vi "Engineering mode.vi"() -> ()   [LabVIEW 2017]
uses:
  Ctrls/TesterInfo.ctl
  Ctrls/control_hard.ctl
  Ctrls/AllControls.ctl
  Ctrls/Position Config.ctl
  Ctrls/HD Config.ctl
  <vilib>/Utility/miscctls.llb/LVRowAndColumnTypeDef.ctl
  ComVIS/Files/Ini/WriteIniFiles_ByVarient.vi
  <vilib>/Utility/file.llb/Write Delimited Spreadsheet (string).vi
  HardWare/ADLINK/IO/Adlink IO/Adlink IO.lvlib
  <instrlib>/GPP/GPP.lvlib
panel:
  out "URAT.COM":refnum<visa-resource-name>
  in  "Production Mode":bool
  out "Boolean":bool=TRUE
  in  "Data":string
  out "Size":i32
  in  "AllControls":T1
  out "Save_status":string
  in  "Selecttion":T2(tab)
  in  "HD Config":T3
  in  "HD Config Save":bool
  in  "SW Config Save":bool
  in  "TesterInfo":T4
  in  "Table":T5(tab)
  in  "Table_Data":string[][](table)
  in  "Title_Data":string[][](table)
  in  "Config":string[][](table)
  in  "SKU_Table":string[][](table)
  in  "Debug":T6
  in  "IO":i32(listbox)
  in  "Reset":bool
  in  "Position Config":T7
  in  "Position Config Save":bool
  in  "NFC":bool
  out "NFC Data":string
  in  "Voltage":dbl min=0.0 max=25.0
  in  "Current":dbl min=0.0 max=48.0
  in  "Read Current&Voltage":bool
  out "ERROR":string
  in  "Write Current&Voltage":bool
  out "Read Current  (A)":dbl
  out "Read Voltage  (V)":dbl
  in  "Set Current  (A)":dbl=1.0
  in  "Set Voltage  (V)":dbl=3.7
  # "Unit: mm"
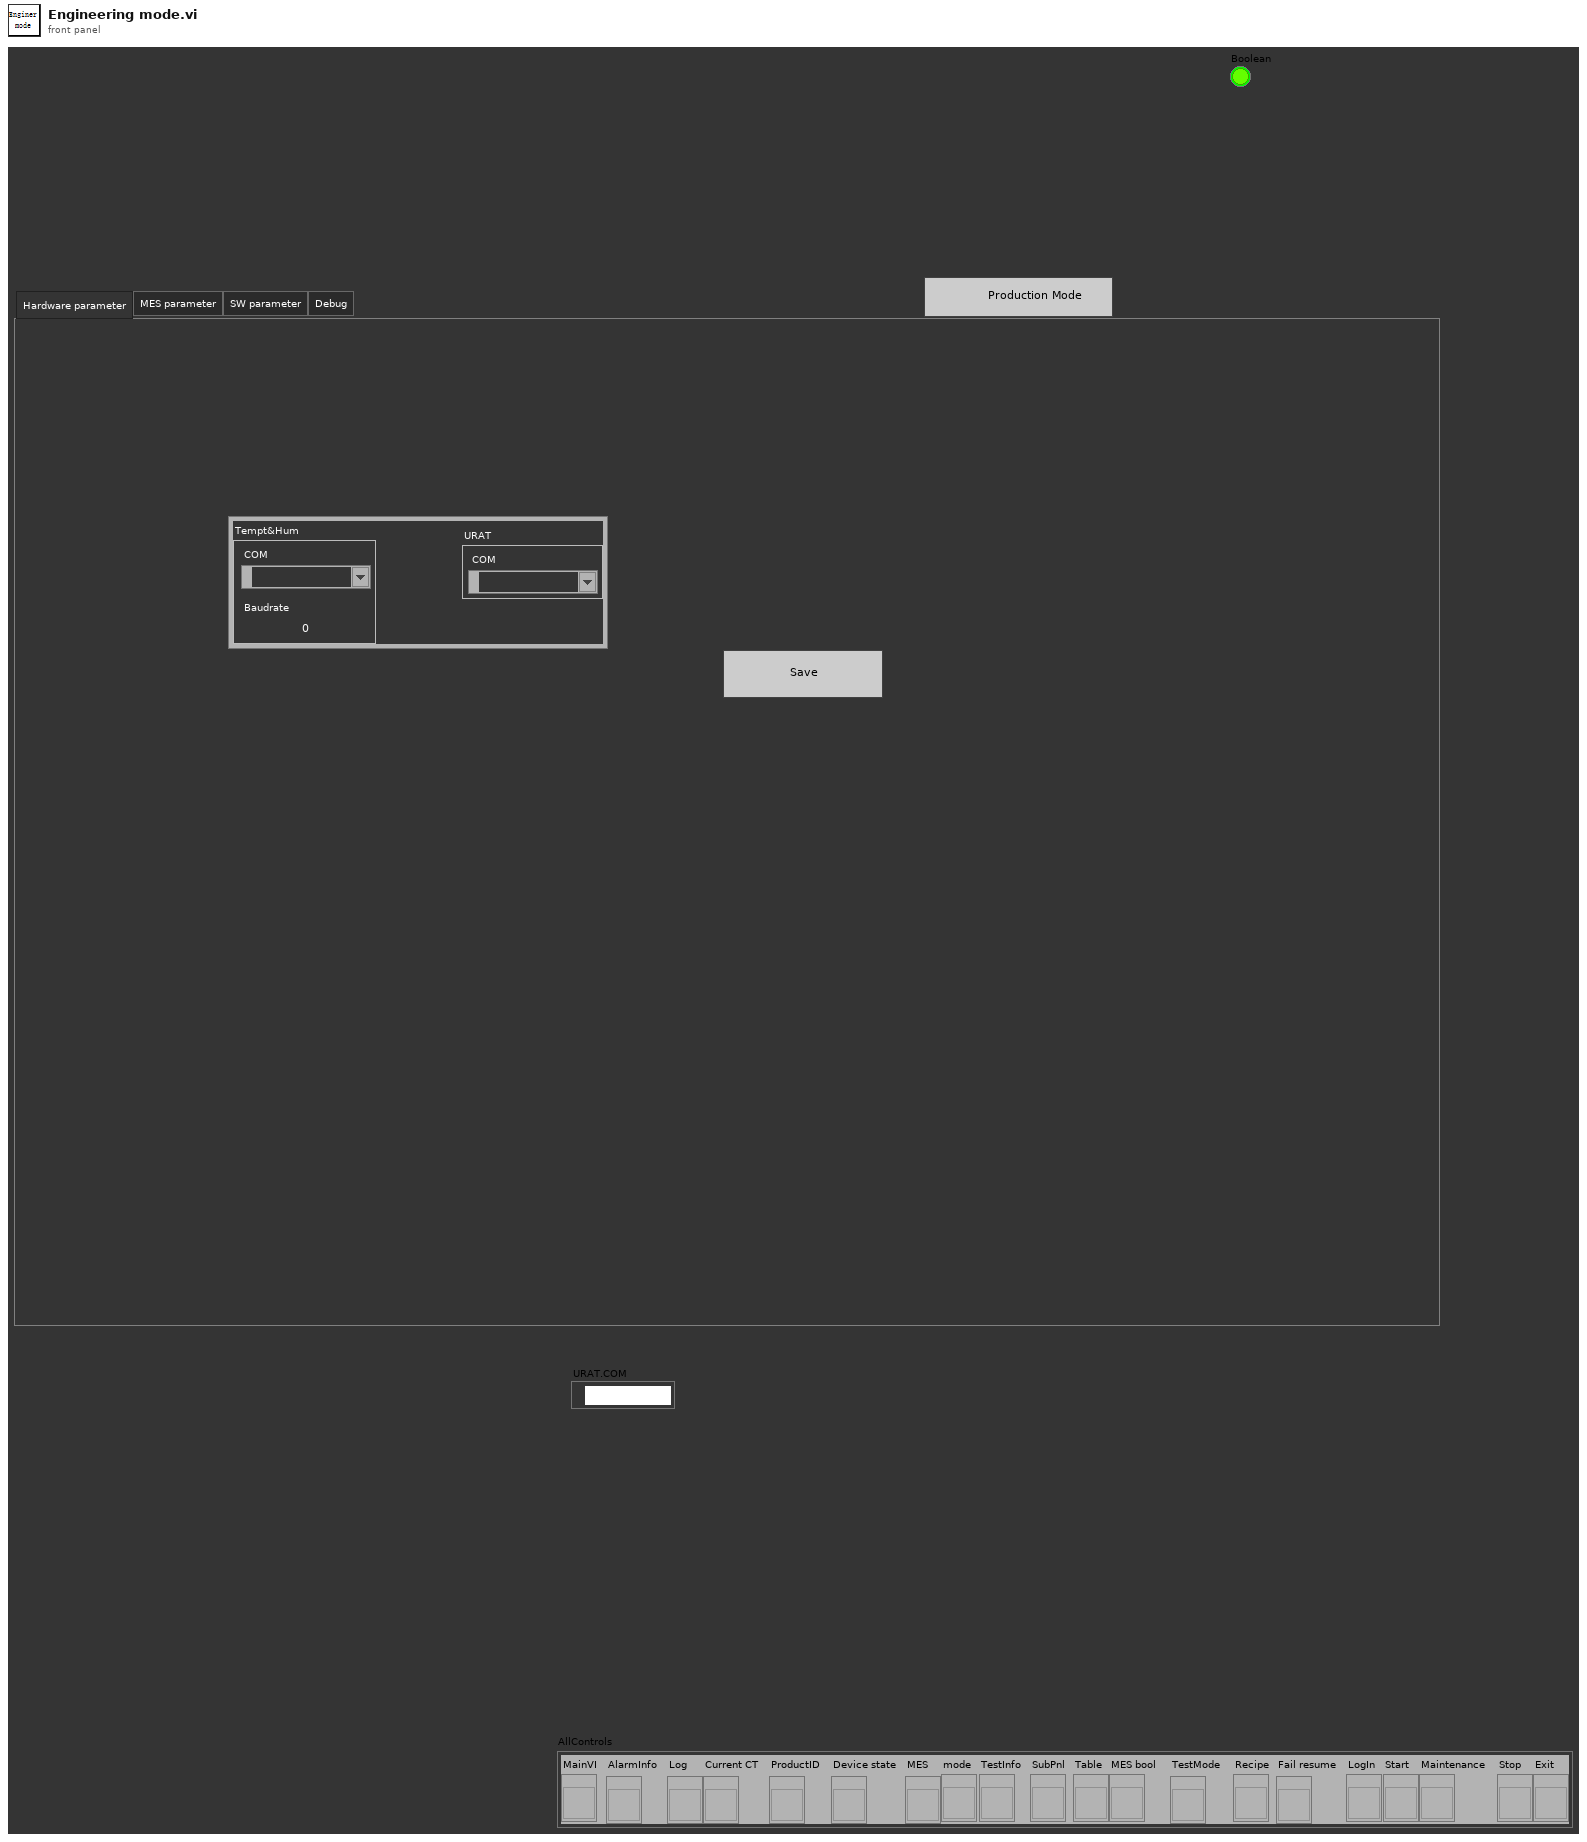
[diagram p1: front panel]
types:
  T1 = typedef "AllControls.ctl" = cluster{"MainVI":refnum<vi>, "AlarmInfo":refnum<vi>, "Log":refnum<vi>, "Current CT":refnum<vi>, "ProductID":refnum<vi>, "Device state":refnum<vi>, "MES":refnum<vi>, "mode":refnum<vi>, "TestInfo":refnum<vi>, "SubPnl":refnum<vi>, "Table":refnum<vi>, "MES bool":refnum<vi>, "TestMode":refnum<vi>, "Recipe":refnum<vi>, "Fail resume":refnum<vi>, "LogIn":refnum<vi>, "Start":refnum<vi>, "Maintenance":refnum<vi>, "Stop":refnum<vi>, "Exit":refnum<vi>}
  T2 = enum32{"Hardware parameter", "MES parameter", "SW parameter", "Debug"}
  T3 = typedef "HD Config.ctl" = cluster{" PC":cluster{"PC Address":u8[], "PC Port":i32}, "FCO":cluster{"COM":refnum<visa-resource-name>, "Baudrate":u32}, "DC Power ":cluster{"COM":refnum<visa-resource-name>, "Baudrate":u32}, "PW3336":cluster{"COM":refnum<visa-resource-name>, "Baudrate":u32}, "Lefoo":cluster{"COM":refnum<visa-resource-name>, "Baudrate":u32}, "Tempt&Hum":cluster{"COM":refnum<visa-resource-name>, "Baudrate":u32}, "DIPC":cluster{"COM":refnum<visa-resource-name>}, "Daemon":cluster{"IP Address":string, "Port":u16, "Retry":u16}, "URAT":cluster{"COM":refnum<visa-resource-name>, "Baudrate":u32}, "Fail_resume_mode":bool, "GRR":bool}
  T4 = typedef "TesterInfo.ctl" = cluster{"Station Name":string, "Station Code":string, "ES NO.":string, "Tester ID":string, "PassMark Revision":string, "Rig ID":string, "Deamon_vision":string, "Project Name":string, "FFTesterPath":path, "Enable_User":bool, "Mode":enum16{"682"}, "MES":bool}
  T5 = enum32{"Process_parameter_Setting", "Passmark_Setting", "Setting_Config", "SKU_Table"}
  T6 = typedef "control_hard.ctl" = enum32{"IO Control", "Motor_Plate control", "Led Read", "NFC ", "PW3336_Power Meter", "Lefoo_Atm Pressure", "Power Supply", "Set EOL_URAT"}
  T7 = typedef "Position Config.ctl" = cluster{"OrificeSize_12.7":i32, "OrificeSize_13":i32, "OrificeSize_30":i32, "OrificeSize_16":i32}
  T8 = cluster{"COM":refnum<visa-resource-name>, "Baudrate":u32}
  T9 = cluster{"DI dev":i32[], "DI line":i32[], "Port":i32[], "DO dev":i32[], "DO line":i32[], "IO Data":string[][], "IO f":i16[]}
  T10 = typedef "amc_Message Queue.ctl" = refnum<queue>
  T11 = typedef "LVRowAndColumnTypeDef.ctl" = cluster{"Row":i32, "Column":i32}
  T12 = typedef "LVPoint32TypeDef.ctl" = cluster{"Horizontal":i32, "Vertical":i32}
  T13 = enum8{"Enabled", "Disabled", "Disabled and Grayed Out"}
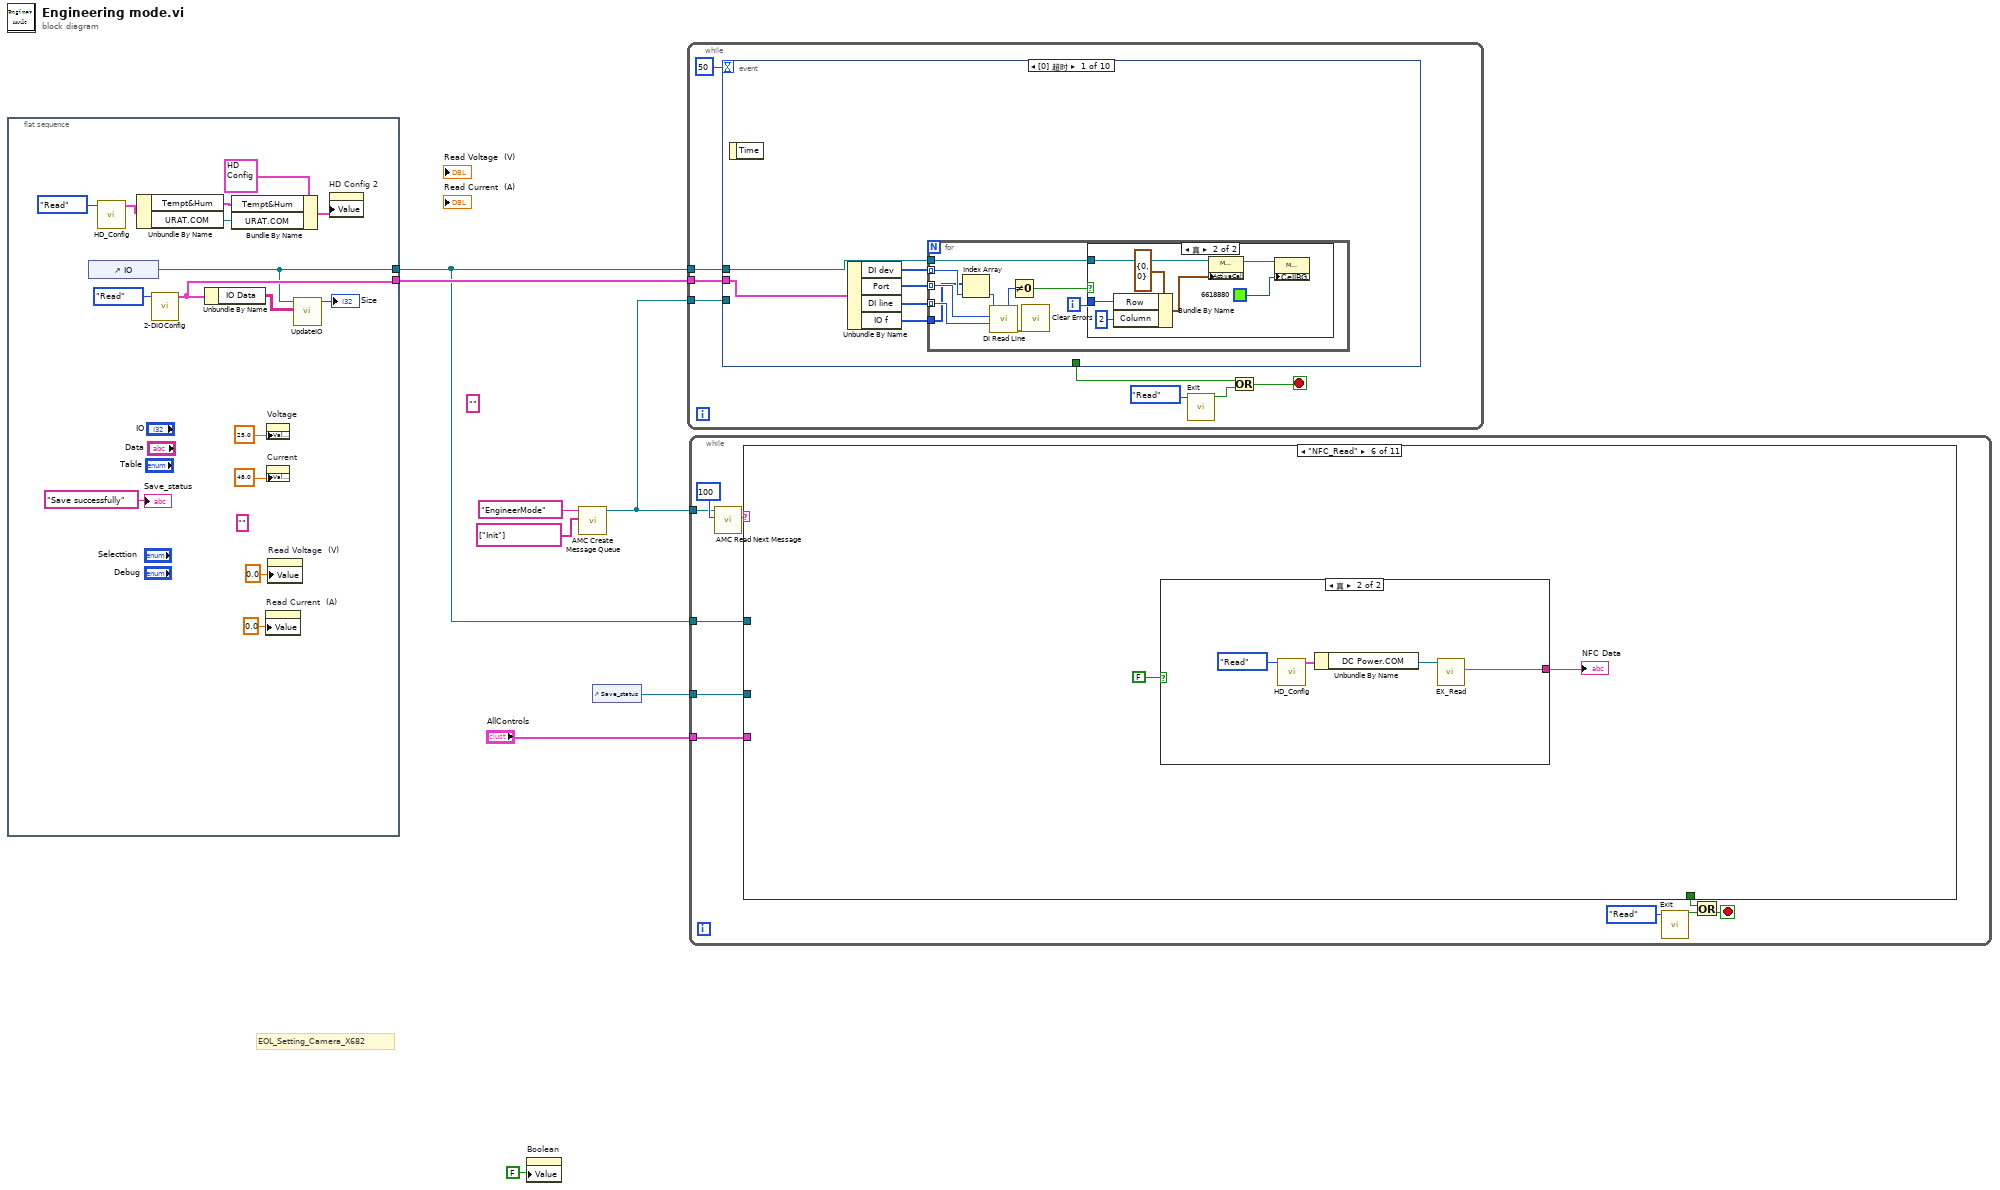
[diagram p0: block diagram]
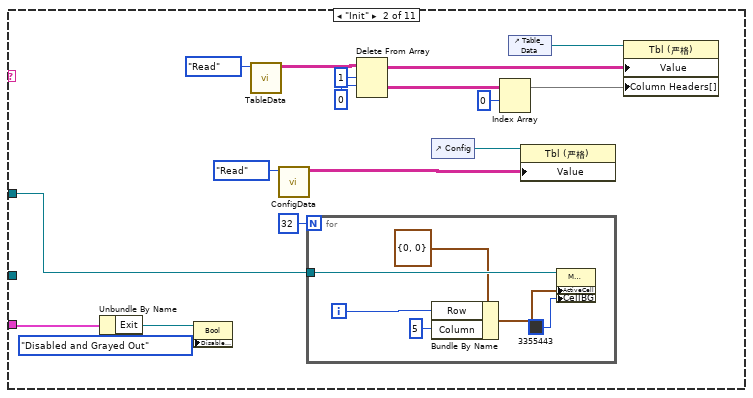
[diagram p3: hidden frame]
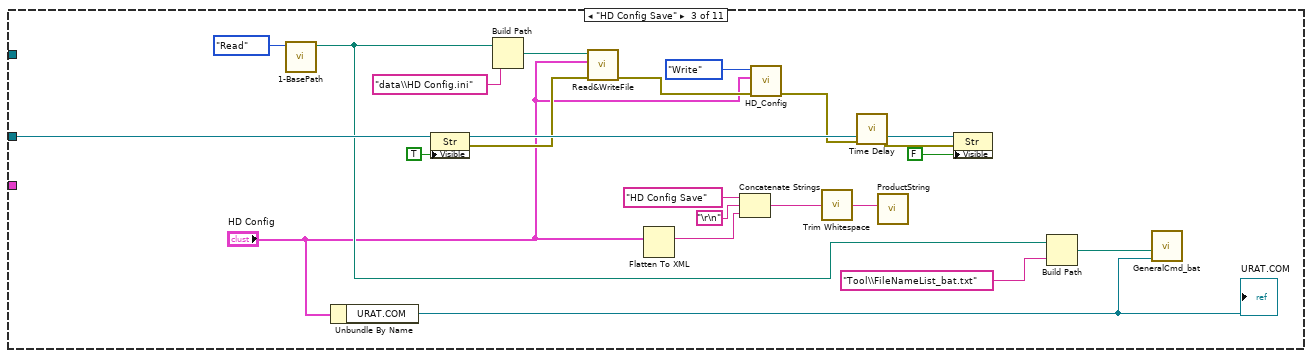
[diagram p4: hidden frame]
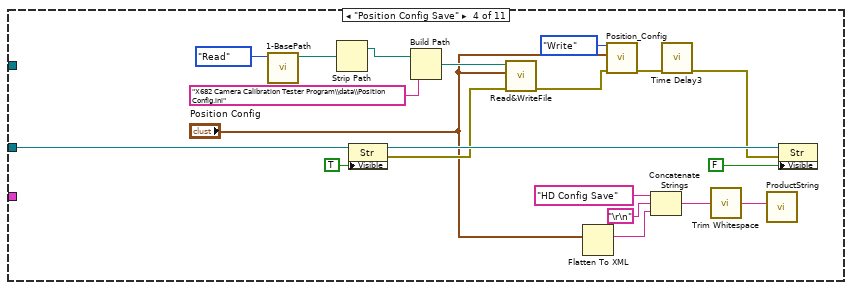
[diagram p5: hidden frame]
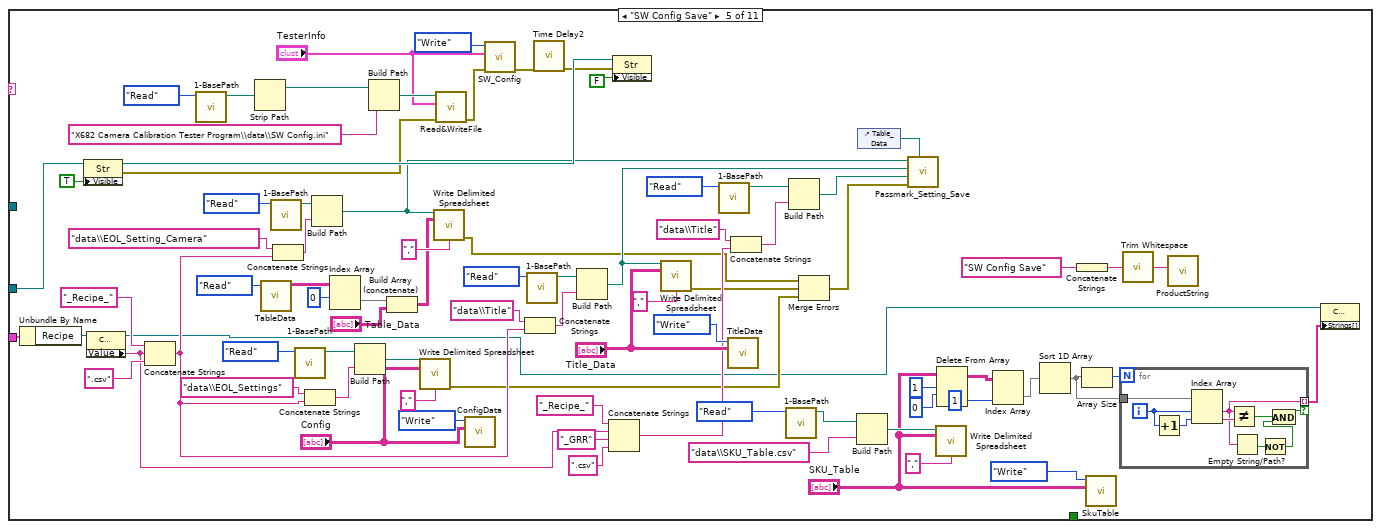
[diagram p6: hidden frame]
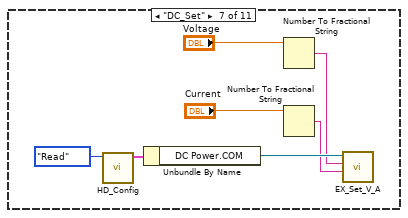
[diagram p8: hidden frame]
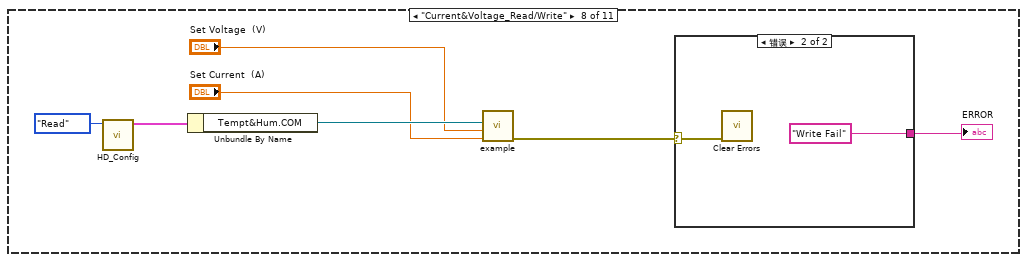
[diagram p9: hidden frame]
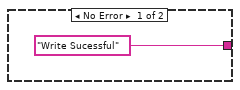
[diagram p10: hidden frame]
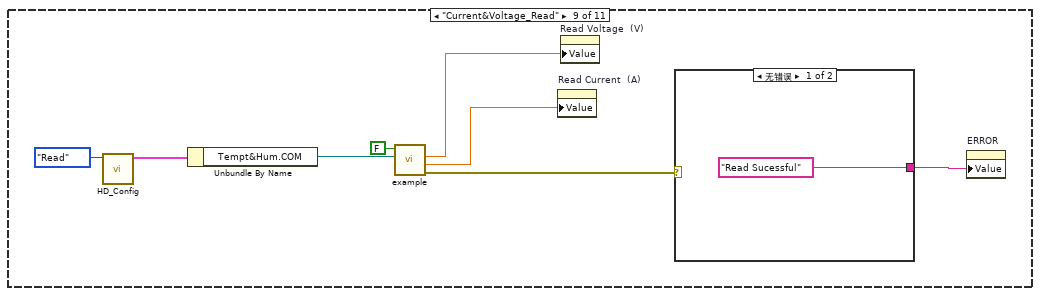
[diagram p11: hidden frame]
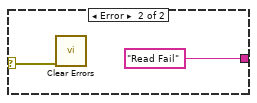
[diagram p12: hidden frame]
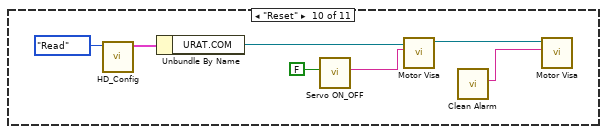
[diagram p13: hidden frame]
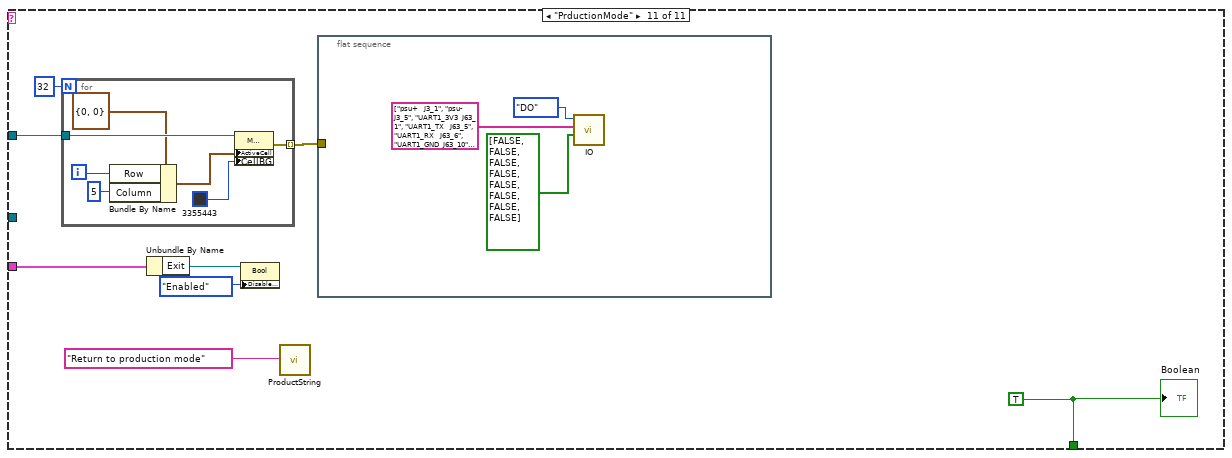
[diagram p14: hidden frame]
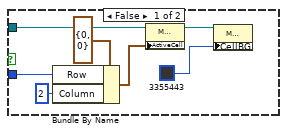
[diagram p15: hidden frame]
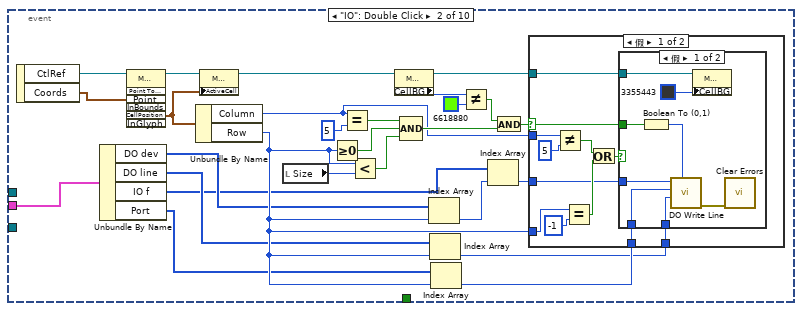
[diagram p16: hidden frame]
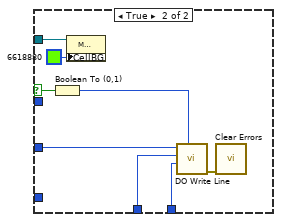
[diagram p18: hidden frame]
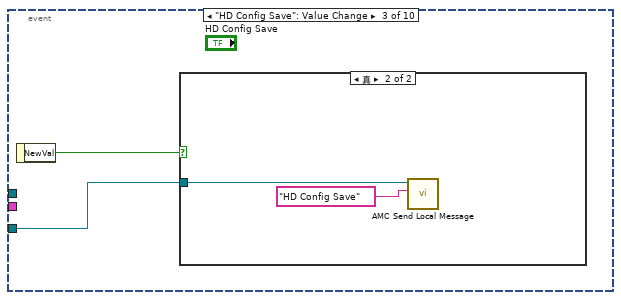
[diagram p19: hidden frame]
diagram:
  (unwired) "" ("concatenated string")
  # "EOL_Setting_Camera_X682"
  n1 = flat-sequence {
    tunnel: [w23] -> w3
    tunnel: [w21] -> w2
    frame #0 {
      (unwired) "" ("Data Return")
      n2 = control-ref of="IO"() -> (w21:refnum<vi>)
      n3 = call "HD_Config.vi"("Step"=enum16{"Initial", "Write", "Read"}."Read") -> ("HD Config out"=w17:T3)  [unwired: 9 in, 1 out]
      n4 = Unbundle By Name(w17) -> ("Tempt&Hum"=w14:T8, "URAT.COM"=w10:refnum<visa-resource-name>)
      n5 = call "2-DIOConfig.vi"("Step"=enum16{"Initial", "Write", "Read"}."Read") -> ("DIO pra out"=w23:T9)  [unwired: 9 in, 1 out]
      n6 = Unbundle By Name(w23) -> ("IO Data"=w22:string[][])
      n7 = Bundle By Name(cluster=T3 {" PC"={"PC Address"=[], "PC Port"=0}, "FCO"={"COM"="", "Baudrate"=0}, "DC Power "={"COM"="", "Baudrate"=0}, "PW3336"={"COM"="", "Baudrate"=0}, "Lefoo"={"COM"="", "Baudrate"=0}, "Tempt&Hum"={"COM"="", "Baudrate"=0}, "DIPC"={"COM"=""}, "Daemon"={"IP Address"="", "Port"=0, "Retry"=0}, "URAT"={"COM"="", "Baudrate"=0}, "Fail_resume_mode"=FALSE, "GRR"=FALSE} ("HD Config 2"), "Tempt&Hum"=w14, "URAT.COM"=w10) -> (w13:T3)
      n8 = property on="Read Current  (A)" class="DigNum (严格)"("Value"=0.0 ("Read Current")) -> ()  [unwired: 2 in, 2 out]
      n9 = property on="Voltage" class="DigNum (strict)"("Value"=25.0 ("Voltage")) -> ()  [unwired: 2 in, 2 out]
      n10 = property on="Current" class="DigNum (strict)"("Value"=48.0 ("Current")) -> ()  [unwired: 2 in, 2 out]
      n11 = property on="Read Voltage  (V)" class="DigNum (严格)"("Value"=0.0 ("Read Voltage")) -> ()  [unwired: 2 in, 2 out]
      n12 = call "UpdateIO.vi"("IO Data"=w22, "MulticolumnListbox输入"=w21) -> ("大小"=→"Size":i32)  [unwired: 9 in]
      n13 = property on="HD Config 2" class="Clust (严格)"("Value"=w13) -> ()  [unwired: 2 in, 2 out]
      "Save_status" <- "Save successfully" ("Save_status")
    }
  }
  n14 = property on="Boolean" class="Bool (严格)"("Value"=FALSE ("Boolean")) -> ()  [unwired: 2 in, 2 out]
  n15 = call "AMC Create Message Queue.vi"("Initial Message Names"=string[] ["Init"], "Message Queue Name"="EngineerMode" ("Message queue name (unnamed)")) -> ("Message Queue out"=w7:T10)  [unwired: 3 in, 6 out]
  n16 = control-ref of="Save_status"() -> (w6:refnum<vi>)
  n17 = while {
    tunnel: w7 -> [w29]
    tunnel: w2 -> [w27]
    tunnel: w3 -> [w26]
    stop <- w25 stop-if-true
    n18 = event shown="[0] 超时" {
      selector: _ -> [_ _ _ _ _ _ _ _ _ _]
      dyn-events: _ -> [_ _ _ _ _ _ _ _ _ _]
      timeout: 50 -> [_ _ _ _ _ _ _ _ _ _]
      tunnel: w29 -> [_ _ w119 w122 w127 w132 w139 w143 w146 w151]
      tunnel: [_ _ _ _ _ _ _ _ _ w150] -> w28
      tunnel: w27 -> [w33 _ _ _ _ _ _ _ _ _]
      tunnel: w26 -> [w34 w65 _ _ _ _ _ _ _ _]
      event Timeout {
        n19 = event-data() -> ()  [unwired: 1 in, 1 out]
        n20 = Unbundle By Name(w34) -> ("DI dev"=w35:i32[], "Port"=w36:i32[], "DI line"=w37:i32[], "IO f"=w38:i16[])
        n21 = for {
          tunnel: w33 -> [w44]
          tunnel: w35 -> [w41] mode=indexing
          tunnel: w37 -> [w45] mode=indexing
          tunnel: w36 -> [w42] mode=indexing
          tunnel: w38 -> [w39]
          i -> [w43]
          n22 = Index Array(array=w39, index=w41) -> (element=w40:i16)
          n23 = call "DI Read Line.vi"("Line"=w45, "Port"=w42, "CardNumber"=w40) -> ("error out"=w48:errorcluster, "State out"=w47:u16)  [unwired: 6 in, 1 out]
          n24 = Not Equal To 0?(x=w47) -> (x != 0?=w46:bool)
          n25 = call <vilib>:"Clear Errors.vi"("error in (no error)"=w48) -> ()  [unwired: 5 in, 2 out]
          n26 = case shown="真" w46 {
            tunnel: w43 -> [w50 w59]
            tunnel: w44 -> [w49 w56]
            frame False {
              n27 = Bundle By Name(cluster=T11 {"Row"=0, "Column"=0} ("活动单元格:活动单元格"), "Row"=w50, "Column"=2) -> (w53:T11)
              n28 = property class="MCListbox (严格)"(reference=w49, "ActiveCell"=w53) -> (reference out=w55:refnum<vi>)  [unwired: 1 in, 1 out]
              n29 = property class="MCListbox (严格)"(reference=w55, "CellBG"=u32 3355443) -> ()  [unwired: 1 in, 2 out]
            }
            frame True {
              n30 = Bundle By Name(cluster=T11 {"Row"=0, "Column"=0} ("活动单元格:活动单元格"), "Row"=w59, "Column"=2) -> (w60:T11)
              n31 = property class="MCListbox (严格)"(reference=w56, "ActiveCell"=w60) -> (reference out=w62:refnum<vi>)  [unwired: 1 in, 1 out]
              n32 = property class="MCListbox (严格)"(reference=w62, "CellBG"=u32 6618880) -> ()  [unwired: 1 in, 2 out]
            }
          }
        }
      }
      event "IO": Double Click {
        n33 = event-data() -> ("CtlRef"=w64:refnum<vi>, "Coords"=w63:T12)  [unwired: 1 in]
        n34 = Unbundle By Name(w65) -> ("DO dev"=w70:i32[], "DO line"=w69:i32[], "IO f"=w68:i16[], "Port"=w87:i32[])
        n35 = invoke class="MCListbox (严格)" method="Point To Row Column"(reference=w64, "Point"=w63) -> (reference out=w83:refnum<vi>, "CellPosition"=w74:T11)  [unwired: 5 in, 5 out]
        n36 = Unbundle By Name(w74) -> ("Column"=w71:i32, "Row"=w88:i32)
        n37 = property class="MCListbox (严格)"(reference=w83, "ActiveCell"=w74) -> (reference out=w82:refnum<vi>)  [unwired: 1 in, 1 out]
        n38 = local read "Size"() -> (w73:i32)
        n39 = Greater Or Equal To 0?(x=w88) -> (x >= 0?=w79:bool)
        n40 = Equal?(x=w71, y=5) -> (x = y?=w80:bool)
        n41 = Less?(x=w88, y=w73) -> (x < y?=w72:bool)
        n42 = property class="MCListbox (严格)"(reference=w82) -> (reference out=w75:refnum<vi>, "CellBG"=w77:u32)  [unwired: 1 in, 1 out]
        n43 = Compound Arithmetic op=AND(w80, w79, w72) -> (w81:bool)
        n44 = Index Array(array=w70, index=w88) -> (element=w84:i32)
        n45 = Index Array(array=w69, index=w88) -> (element=w86:i32)
        n46 = Index Array(array=w87, index=w88) -> (element=w89:i32)
        n47 = Not Equal?(x=w77, y=u32 6618880) -> (x != y?=w78:bool)
        n48 = Index Array(array=w68, index=w84) -> (element=w85:i16)
        n49 = And(x=w78, y=w81) -> (x .and. y?=w76:bool)
        n50 = case shown="假" w76 {
          selector: w76 -> [w98 w113]
          tunnel: w75 -> [w101 w117]
          tunnel: w71 -> [w97 _]
          tunnel: w85 -> [w92 w115]
          tunnel: w86 -> [w91 w114]
          tunnel: w88 -> [w93 _]
          tunnel: w89 -> [w90 w110]
          frame False {
            n51 = Not Equal?(x=w97, y=5) -> (x != y?=w94:bool)
            n52 = Equal?(x=w93, y=-1) -> (x = y?=w99:bool)
            n53 = Or(x=w94, y=w99) -> (x .or. y?=w95:bool)
            n54 = case shown="假" w95 {
              tunnel: w101 -> [w108 _]
              tunnel: w98 -> [w103 _]
              tunnel: w92 -> [w104 _]
              tunnel: w91 -> [w105 _]
              tunnel: w90 -> [w102 _]
              frame False {
                n55 = Boolean To (0,1)(Boolean=w103) -> (0, 1=w107:i16)
                n56 = call "DO Write Line.vi"("Value"=w107, "Line"=w105, "Port"=w102, "CardNumber"=w104) -> ("error out"=w106:errorcluster)  [unwired: 6 in, 1 out]
                n57 = property class="MCListbox (严格)"(reference=w108, "CellBG"=u32 3355443) -> ()  [unwired: 1 in, 2 out]
                n58 = call <vilib>:"Clear Errors.vi"("error in (no error)"=w106) -> ()  [unwired: 5 in, 2 out]
              }
              frame True {
              }
            }
          }
          frame True {
            n59 = Boolean To (0,1)(Boolean=w113) -> (0, 1=w112:i16)
            n60 = property class="MCListbox (严格)"(reference=w117, "CellBG"=u32 6618880) -> ()  [unwired: 1 in, 2 out]
            n61 = call "DO Write Line.vi"("Value"=w112, "Line"=w114, "Port"=w110, "CardNumber"=w115) -> ("error out"=w111:errorcluster)  [unwired: 6 in, 1 out]
            n62 = call <vilib>:"Clear Errors.vi"("error in (no error)"=w111) -> ()  [unwired: 5 in, 2 out]
          }
        }
      }
      event "HD Config Save": Value Change {
        n63 = event-data() -> ("NewVal"=w118:bool)  [unwired: 1 in]
        n64 = case shown="真" w118 {
          tunnel: w119 -> [_ w121]
          frame False {
          }
          frame True {
            n65 = call "AMC Send Local Message.vi"("Message Name"="HD Config Save", "Message Queue in"=w121) -> ()  [unwired: 8 in, 2 out]
          }
        }
      }
      event "SW Config Save": Value Change {
        n66 = event-data() -> ("NewVal"=w123:bool)  [unwired: 1 in]
        n67 = case shown="真" w123 {
          tunnel: w122 -> [_ w125]
          frame False {
          }
          frame True {
            n68 = call "AMC Send Local Message.vi"("Message Name"="SW Config Save", "Message Queue in"=w125) -> ()  [unwired: 8 in, 2 out]
          }
        }
      }
      event "Position Config Save": Value Change {
        n69 = event-data() -> ("NewVal"=w126:bool)  [unwired: 1 in]
        n70 = case shown="真" w126 {
          tunnel: w127 -> [_ w129]
          frame False {
          }
          frame True {
            n71 = call "AMC Send Local Message.vi"("Message Name"="Position Config Save", "Message Queue in"=w129) -> ()  [unwired: 8 in, 2 out]
          }
        }
      }
      event "Write Current&Voltage": Value Change {
        n72 = event-data() -> ("NewVal"=w131:bool)  [unwired: 1 in]
        n73 = case shown="真" w131 {
          tunnel: w132 -> [_ w133]
          frame False {
          }
          frame True {
            n74 = call "AMC Send Local Message.vi"("Message Name"="Current&Voltage_Read/Write", "Message Queue in"=w133) -> ()  [unwired: 8 in, 2 out]
          }
        }
        n75 = property on="ERROR" class="Str"("Value"="" ("ERROR")) -> ()  [unwired: 2 in, 2 out]
      }
      event "Read Current&Voltage": Value Change {
        n76 = event-data() -> ("NewVal"=w138:bool)  [unwired: 1 in]
        n77 = case shown="真" w138 {
          tunnel: w139 -> [_ w140]
          frame False {
          }
          frame True {
            n78 = call "AMC Send Local Message.vi"("Message Name"="Current&Voltage_Read", "Message Queue in"=w140) -> ()  [unwired: 8 in, 2 out]
          }
        }
        n79 = property on="ERROR" class="Str"("Value"="" ("ERROR")) -> ()  [unwired: 2 in, 2 out]
        n80 = property on="Read Current  (A)" class="DigNum (严格)"("Value"=0.0 ("Read Current")) -> ()  [unwired: 2 in, 2 out]
        n81 = property on="Read Voltage  (V)" class="DigNum (严格)"("Value"=0.0 ("Read Voltage")) -> ()  [unwired: 2 in, 2 out]
      }
      event "NFC": Value Change {
        n82 = event-data() -> ("NewVal"=w142:bool)  [unwired: 1 in]
        n83 = case shown="真" w142 {
          tunnel: w143 -> [_ w144]
          frame False {
          }
          frame True {
            n84 = call "AMC Send Local Message.vi"("Message Name"="NFC_Read", "Message Queue in"=w144) -> ()  [unwired: 8 in, 2 out]
          }
        }
      }
      event "Reset": Value Change {
        n85 = event-data() -> ("NewVal"=w147:bool)  [unwired: 1 in]
        n86 = case shown="真" w147 {
          tunnel: w146 -> [_ w149]
          frame False {
          }
          frame True {
            n87 = call "AMC Send Local Message.vi"("Message Name"="Reset", "Message Queue in"=w149) -> ()  [unwired: 8 in, 2 out]
          }
        }
      }
      event "Production Mode": Value Change {
        n88 = event-data() -> ("NewVal"=w152:bool)  [unwired: 1 in]
        n89 = case shown="真" w152 {
          tunnel: w151 -> [_ w154]
          tunnel: [_ TRUE ("停止")] -> w150
          frame False {
          }
          frame True {
            n90 = call "AMC Send Local Message.vi"("Message Name"="PrductionMode", "Message Queue in"=w154) -> ()  [unwired: 8 in, 2 out]
          }
        }
      }
    }
    n91 = call "Exit.vi"("Step"=enum16{"Initial", "Write", "Read"}."Read") -> ("Exit Out"=w31:bool)  [unwired: 9 in, 1 out]
    n92 = Or(x=w28, y=w31) -> (x .or. y?=w25:bool)
  }
  n93 = while {
    tunnel: w7 -> [w162]
    tunnel: w6 -> [w158]
    tunnel: "AllControls" -> [w157]
    tunnel: w2 -> [w156]
    stop <- w160 stop-if-true
    n94 = call "AMC Read Next Message.vi"("timeout (1ms)"=100 ("Timeout"), "Message Queue in"=w162) -> ("Message Name"=w161:string)  [unwired: 2 in, 7 out]
    n95 = case shown="\"NFC_Read\"" w161 {
      tunnel: [_ _ _ _ _ _ _ _ _ _ w370] -> w159
      tunnel: w158 -> [_ _ w202 w221 w309 _ _ _ _ _ _]
      tunnel: w157 -> [_ w168 _ _ w276 _ _ _ _ _ w364]
      tunnel: w156 -> [_ w169 _ _ _ _ _ _ _ _ w369]
      frame "假", Default {
      }
      frame "Init" {
        n96 = Unbundle By Name(w168) -> ("Exit"=w167:refnum<vi>)
        n97 = property class="Bool"(reference=w167, "DisabledEnum"=T13."Disabled and Grayed Out" ("Disabled")) -> ()  [unwired: 1 in, 2 out]
        n98 = call "TableData.vi"("Step"=enum16{"Initial", "Write", "Read"}."Read") -> ("Tabledata Out"=w178:string[][])  [unwired: 9 in, 1 out]
        n99 = call "ConfigData.vi"("Step"=enum16{"Initial", "Write", "Read"}."Read") -> ("Tabledata Out"=w171:string[][])  [unwired: 9 in, 1 out]
        n100 = for {
          N: 32 -> [_]
          tunnel: w169 -> [w188]
          i -> [w184]
          n101 = Bundle By Name(cluster=T11 {"Row"=0, "Column"=0} ("Active Cell:Active Cell"), "Row"=w184, "Column"=5) -> (w185:T11)
          n102 = property class="MCListbox (严格)"(reference=w188, "ActiveCell"=w185, "CellBG"=u32 3355443) -> ()  [unwired: 1 in, 2 out]
        }
        n103 = Delete From Array(array=w178, length=1 ("长度"), index (row)=0 ("索引 (行)")) -> (deleted portion=w176:string[][], array with subset deleted=w177:string[][])  [unwired: 1 in]
        n104 = control-ref of="Config"() -> (w172:refnum<vi>)
        n105 = Index Array(array=w176, index (row)=0 ("索引 (行)")) -> (element=w175:string[])  [unwired: 1 in]
        n106 = control-ref of="Table_Data"() -> (w182:refnum<vi>)
        n107 = property on="属性节点" class="Tbl (严格)"(reference=w172, "Value"=w171) -> ()  [unwired: 1 in, 2 out]
        n108 = property on="属性节点" class="Tbl (严格)"(reference=w182, "Value"=w177, "Column Headers[]"=w175) -> ()  [unwired: 1 in, 2 out]
      }
      frame "HD Config Save" {
        n109 = call "1-BasePath.vi"("Step"=enum16{"Initial", "Write", "Read"}."Read") -> ("Path Out"=w191:path)  [unwired: 9 in, 1 out]
        n110 = Unbundle By Name("HD Config") -> ("URAT.COM"=w189:refnum<visa-resource-name>)
        "URAT.COM" <- w189
        n111 = property class="Str"(reference=w202, "Visible"=TRUE ("可见")) -> (reference out=w205:refnum<vi>, error out=w204:errorcluster)  [unwired: 1 in]
        n112 = Build Path(base path=w191, name or relative path="data\\HD Config.ini") -> (appended path=w208:path)
        n113 = call-poly "Read&WriteFile.vi"("error in (no error)"=w204, "Variant"="HD Config", "path"=w208) -> ("error out"=w195:errorcluster)  [unwired: 8 in]
        n114 = Flatten To XML(anything="HD Config") -> (xml string=w200:string)
        n115 = Concatenate Strings("HD Config Save" ("String"), "\r\n", w200) -> (w201:string)
        n116 = call "HD_Config.vi"("error in (no error)"=w195, "HD Config in"="HD Config", "Step"=enum16{"Initial", "Write", "Read"}."Write") -> ("error out"=w194:errorcluster)  [unwired: 7 in, 1 out]
        n117 = call <vilib>:"Trim Whitespace.vi"("string"=w201) -> ("trimmed string"=w198:string)  [unwired: 1 in]
        n118 = call "Time Delay"("error in (no error)"=w194) -> ("error out"=w196:errorcluster)  [unwired: 10 in]
        n119 = call "ProductString.vi"("String"=w198) -> ()  [unwired: 10 in, 1 out]
        n120 = property class="Str"(reference=w205, error in=w196, "Visible"=FALSE ("可见")) -> ()  [unwired: 2 out]
        n121 = Build Path(base path=w191, name or relative path="Tool\\FileNameList_bat.txt") -> (appended path=w193:path)
        n122 = call "GeneralCmd_bat.vi"("COM"=w189, "fileList_bat"=w193) -> ()  [unwired: 9 in, 1 out]
      }
      frame "Position Config Save" {
        n123 = call "1-BasePath.vi"("Step"=enum16{"Initial", "Write", "Read"}."Read") -> ("Path Out"=w229:path)  [unwired: 9 in, 1 out]
        n124 = Strip Path(path=w229) -> (stripped path=w211:path)  [unwired: 1 out]
        n125 = property class="Str"(reference=w221, "Visible"=TRUE ("可见")) -> (reference out=w224:refnum<vi>, error out=w223:errorcluster)  [unwired: 1 in]
        n126 = Build Path(base path=w211, name or relative path="X682 Camera Calibration Tester Program\\data\\Position Config.ini") -> (appended path=w227:path)
        n127 = call-poly "Read&WriteFile.vi"("error in (no error)"=w223, "Variant"="Position Config", "path"=w227) -> ("error out"=w214:errorcluster)  [unwired: 8 in]
        n128 = Flatten To XML(anything="Position Config") -> (xml string=w219:string)
        n129 = call "Position_Config.vi"("error in (no error)"=w214, "Position Config"="Position Config", "Step"=enum16{"Initial", "Write", "Read"}."Write") -> ("error out"=w213:errorcluster)  [unwired: 7 in, 1 out]
        n130 = Concatenate Strings("HD Config Save" ("String"), "\r\n", w219) -> (w220:string)
        n131 = call "Time Delay3"("error in (no error)"=w213) -> ("error out"=w212:errorcluster)  [unwired: 10 in]
        n132 = call <vilib>:"Trim Whitespace.vi"("string"=w220) -> ("trimmed string"=w217:string)  [unwired: 1 in]
        n133 = call "ProductString.vi"("String"=w217) -> ()  [unwired: 10 in, 1 out]
        n134 = property class="Str"(reference=w224, error in=w212, "Visible"=FALSE ("可见")) -> ()  [unwired: 2 out]
      }
      frame "SW Config Save" {
        n135 = Unbundle By Name(w276) -> ("Recipe"=w236:refnum<vi>)
        n136 = property class="Str"(reference=w309, "Visible"=TRUE ("可见")) -> (reference out=w311:refnum<vi>, error out=w301:errorcluster)  [unwired: 1 in]
        n137 = property class="CmbBox"(reference=w236) -> (reference out=w235:refnum<vi>, "Value"=w258:string)  [unwired: 1 in, 1 out]
        n138 = Concatenate Strings("_Recipe_" ("字符串"), w258, ".csv" ("字符串")) -> (w267:string)
        n139 = call "1-BasePath.vi"("Step"=enum16{"Initial", "Write", "Read"}."Read") -> ("Path Out"=w249:path)  [unwired: 9 in, 1 out]
        n140 = Strip Path(path=w249) -> (stripped path=w248:path)  [unwired: 1 out]
        n141 = call "TableData.vi"("Step"=enum16{"Initial", "Write", "Read"}."Read") -> ("Tabledata Out"=w291:string[][])  [unwired: 9 in, 1 out]
        n142 = call "1-BasePath.vi"("Step"=enum16{"Initial", "Write", "Read"}."Read") -> ("Path Out"=w297:path)  [unwired: 9 in, 1 out]
        n143 = Concatenate Strings("data\\EOL_Setting_Camera" ("name or relative path"), w267) -> (w272:string)
        n144 = call "1-BasePath.vi"("Step"=enum16{"Initial", "Write", "Read"}."Read") -> ("Path Out"=w285:path)  [unwired: 9 in, 1 out]
        n145 = Concatenate Strings("data\\EOL_Settings" ("name or relative path"), w267) -> (w270:string)
        n146 = Build Path(base path=w297, name or relative path=w272) -> (appended path=w266:path)
        n147 = Index Array ("索引数组")(array=w291, index (row)=0 ("索引 (行)")) -> (element=w290:string[])  [unwired: 1 in]
        n148 = Build Path(base path=w285, name or relative path=w270) -> (appended path=w287:path)
        n149 = Build Path(base path=w248, name or relative path="X682 Camera Calibration Tester Program\\data\\SW Config.ini") -> (appended path=w303:path)
        n150 = Build Array (concatenate)(w290, "Table_Data") -> (w294:string[][])
        n151 = call-poly <vilib>:"Write Delimited Spreadsheet.vi"("file path (dialog if empty)"=w287, "2D data"="Config", "delimiter (\\t)"="," ("delimiter (\\t)")) -> ("error out"=w251:errorcluster)  [unwired: 11 in, 1 out]
        n152 = call-poly <vilib>:"Write Delimited Spreadsheet.vi"("file path (dialog if empty)"=w266, "2D data"=w294, "delimiter (\\t)"="," ("delimiter (\\t)")) -> ("error out"=w250:errorcluster)  [unwired: 11 in, 1 out]
        n153 = call-poly "Read&WriteFile.vi"("error in (no error)"=w301, "Variant"="TesterInfo", "path"=w303) -> ("error out"=w300:errorcluster)  [unwired: 8 in]
        n154 = call "ConfigData.vi"("Tabledata in"="Config", "Step"=enum16{"Initial", "Write", "Read"}."Write") -> ()  [unwired: 8 in, 2 out]
        n155 = call "SW_Config.vi"("error in (no error)"=w300, "SW Config In"="TesterInfo", "Step"=enum16{"Initial", "Write", "Read"}."Write") -> ("error out"=w299:errorcluster)  [unwired: 7 in, 1 out]
        n156 = Concatenate Strings("data\\Title" ("name or relative path"), w267) -> (w268:string)
        n157 = call "1-BasePath.vi"("Step"=enum16{"Initial", "Write", "Read"}."Read") -> ("Path Out"=w279:path)  [unwired: 9 in, 1 out]
        n158 = call "Time Delay2"("error in (no error)"=w299) -> ("error out"=w283:errorcluster)  [unwired: 10 in]
        n159 = Build Path(base path=w279, name or relative path=w268) -> (appended path=w265:path)
        n160 = Concatenate Strings("_Recipe_" ("字符串"), w258, "_GRR" ("字符串"), ".csv" ("字符串")) -> (w255:string)
        n161 = property class="Str"(reference=w311, error in=w283, "Visible"=FALSE ("可见")) -> ()  [unwired: 2 out]
        n162 = call-poly <vilib>:"Write Delimited Spreadsheet.vi"("file path (dialog if empty)"=w265, "2D data"="Title_Data", "delimiter (\\t)"="," ("delimiter (\\t)")) -> ("error out"=w254:errorcluster)  [unwired: 11 in, 1 out]
        n163 = call "1-BasePath.vi"("Step"=enum16{"Initial", "Write", "Read"}."Read") -> ("Path Out"=w262:path)  [unwired: 9 in, 1 out]
        n164 = call "TitleData.vi"("Tabledata in"="Title_Data", "Step"=enum16{"Initial", "Write", "Read"}."Write") -> ()  [unwired: 8 in, 2 out]
        n165 = Concatenate Strings("data\\Title" ("name or relative path"), w255) -> (w264:string)
        n166 = call "1-BasePath.vi"("Step"=enum16{"Initial", "Write", "Read"}."Read") -> ("Path Out"=w242:path)  [unwired: 9 in, 1 out]
        n167 = Build Path(base path=w262, name or relative path=w264) -> (appended path=w260:path)
        n168 = Merge Errors(w250, w254, w251) -> (w252:errorcluster)
        n169 = Build Path(base path=w242, name or relative path="data\\SKU_Table.csv") -> (appended path=w247:path)
        n170 = control-ref of="Table_Data"() -> (w253:refnum<vi>)
        n171 = call "Passmark_Setting_Save.vi"("Table_Data 2"=w253, "error in (no error)"=w252, "GRR_Title_Setting_path"=w260, "Title_Setting_path"=w265, "Flow_Setting_path"=w266) -> ()  [unwired: 6 in, 1 out]
        n172 = call-poly <vilib>:"Write Delimited Spreadsheet.vi"("file path (dialog if empty)"=w247, "2D data"="SKU_Table", "delimiter (\\t)"="," ("delimiter (\\t)")) -> ()  [unwired: 11 in, 2 out]
        n173 = Delete From Array(array="SKU_Table", length=1 ("长度"), index (row)=0 ("索引 (行)")) -> (array with subset deleted=w241:string[][])  [unwired: 1 in, 1 out]
        n174 = Index Array(array=w241, index (col)=1 ("禁用的索引 (列)")) -> (element=w234:string[])  [unwired: 1 in]
        n175 = Sort 1D Array(array=w234) -> (sorted array=w232:string[])
        n176 = Concatenate Strings("SW Config Save" ("String")) -> (w308:string)
        n177 = Array Size(array=w232) -> (size(s)=w233:i32)
        n178 = call "SkuTable.vi"("Tabledata in"="SKU_Table", "Step"=enum16{"Initial", "Write", "Read"}."Write") -> ()  [unwired: 8 in, 2 out]
        n179 = for {
          N: w233 -> [_]
          tunnel: w232 -> [w321]
          tunnel: [w316] -> w231 mode=indexing if=w314
          i -> [w319]
          n180 = Increment(x=w319) -> (x+1=w318:i32)
          n181 = Index Array(array=w321, index #1=w319, index #2=w318) -> (element #1=w316:string, element #2=w317:string)
          n182 = Not Equal?(x=w316, y=w317) -> (x != y?=w320:bool)
          n183 = Empty String/Path?(string/path=w316) -> (empty?=w315:bool)
          n184 = Not(x=w315) -> (.not. x?=w313:bool)
          n185 = And(x=w320, y=w313) -> (x .and. y?=w314:bool)
        }
        n186 = call <vilib>:"Trim Whitespace.vi"("string"=w308) -> ("trimmed string"=w307:string)  [unwired: 1 in]
        n187 = call "ProductString.vi"("String"=w307) -> ()  [unwired: 10 in, 1 out]
        n188 = property class="CmbBox"(reference=w235, "Strings[]"=w231) -> ()  [unwired: 1 in, 2 out]
      }
      frame "NFC_Read" {
        n189 = case shown="真" FALSE {
          tunnel: [_ w325] -> w323
          frame False {
          }
          frame True {
            n190 = call "HD_Config.vi"("Step"=enum16{"Initial", "Write", "Read"}."Read") -> ("HD Config out"=w327:T3)  [unwired: 9 in, 1 out]
            n191 = Unbundle By Name(w327) -> ("DC Power.COM"=w324:refnum<visa-resource-name>)
            n192 = call "EX_Read.vi"("VISA resource name"=w324) -> ("读取缓冲区"=w325:string)  [unwired: 8 in, 2 out]
          }
        }
        "NFC Data" <- w323
      }
      frame "DC_Set" {
        n193 = call "HD_Config.vi"("Step"=enum16{"Initial", "Write", "Read"}."Read") -> ("HD Config out"=w334:T3)  [unwired: 9 in, 1 out]
        n194 = Unbundle By Name(w334) -> ("DC Power.COM"=w332:refnum<visa-resource-name>)
        n195 = Number To Fractional String(number="Voltage") -> (F-format string=w331:string)  [unwired: 3 in]
        n196 = Number To Fractional String(number="Current") -> (F-format string=w330:string)  [unwired: 3 in]
        n197 = call "EX_Set_V_A.vi"("current"=w330, "voltage"=w331, "VISA resource name"=w332) -> ()  [unwired: 7 in, 2 out]
      }
      frame "Current&Voltage_Read/Write" {
        n198 = call "HD_Config.vi"("Step"=enum16{"Initial", "Write", "Read"}."Read") -> ("HD Config out"=w341:T3)  [unwired: 9 in, 1 out]
        n199 = Unbundle By Name(w341) -> ("Tempt&Hum.COM"=w339:refnum<visa-resource-name>)
        n200 = call <instrlib>:"example.vi"("Current Level (A)"="Set Current  (A)", "Voltage Level (V)"="Set Voltage  (V)", "VISA resource name"=w339) -> ("error out"=w335:errorcluster)  [unwired: 5 in, 3 out]
        n201 = case shown="错误" w335 {
          selector: w335 -> [_ w343]
          tunnel: ["Write Sucessful" ("ERROR") "Write Fail" ("ERROR")] -> w336
          frame No Error {
          }
          frame Error {
            n202 = call <vilib>:"Clear Errors.vi"("error in (no error)"=w343) -> ()  [unwired: 5 in, 2 out]
          }
        }
        "ERROR" <- w336
      }
      frame "Current&Voltage_Read" {
        n203 = call "HD_Config.vi"("Step"=enum16{"Initial", "Write", "Read"}."Read") -> ("HD Config out"=w352:T3)  [unwired: 9 in, 1 out]
        n204 = Unbundle By Name(w352) -> ("Tempt&Hum.COM"=w350:refnum<visa-resource-name>)
        n205 = call <instrlib>:"example.vi"("VISA resource name"=w350, "FLAG"=FALSE) -> ("error out"=w349:errorcluster, "Actual Current Level (A)"=w345:dbl, "Actual Voltage Level (V)"=w346:dbl)  [unwired: 6 in, 1 out]
        n206 = property on="Read Current  (A)" class="DigNum (严格)"("Value"=w345) -> ()  [unwired: 2 in, 2 out]
        n207 = property on="Read Voltage  (V)" class="DigNum (严格)"("Value"=w346) -> ()  [unwired: 2 in, 2 out]
        n208 = case shown="无错误" w349 {
          selector: w349 -> [_ w354]
          tunnel: ["Read Sucessful" ("ERROR") "Read Fail" ("ERROR")] -> w348
          frame No Error {
          }
          frame Error {
            n209 = call <vilib>:"Clear Errors.vi"("error in (no error)"=w354) -> ()  [unwired: 5 in, 2 out]
          }
        }
        n210 = property on="ERROR" class="Str"("Value"=w348) -> ()  [unwired: 2 in, 2 out]
      }
      frame "Reset" {
        n211 = call "HD_Config.vi"("Step"=enum16{"Initial", "Write", "Read"}."Read") -> ("HD Config out"=w362:T3)  [unwired: 9 in, 1 out]
        n212 = Unbundle By Name(w362) -> ("URAT.COM"=w357:refnum<visa-resource-name>)
        n213 = call "Servo ON_OFF.vi"("Servo ON/OFF"=FALSE) -> ("Command"=w358:string)  [unwired: 10 in]
        n214 = call "Motor Visa.vi"("Command"=w358, "VISA资源名称"=w357) -> ("VISA资源名称输出"=w356:refnum<visa-resource-name>)  [unwired: 7 in, 2 out]
        n215 = call "Clean Alarm.vi"() -> ("Clean Alarm"=w360:string)  [unwired: 11 in]
        n216 = call "Motor Visa.vi"("Command"=w360, "VISA资源名称"=w356) -> ()  [unwired: 7 in, 3 out]
      }
      frame "PrductionMode" {
        w370 = TRUE
        n217 = for {
          N: 32 -> [_]
          tunnel: w369 -> [w377]
          tunnel: [w371] -> w363 mode=indexing
          i -> [w373]
          n218 = Bundle By Name(cluster=T11 {"Row"=0, "Column"=0} ("Active Cell:Active Cell"), "Row"=w373, "Column"=5) -> (w374:T11)
          n219 = property class="MCListbox (严格)"(reference=w377, "ActiveCell"=w374, "CellBG"=u32 3355443) -> (error out=w371:errorcluster)  [unwired: 1 in, 1 out]
        }
        n220 = Unbundle By Name(w364) -> ("Exit"=w366:refnum<vi>)
        n221 = property class="Bool"(reference=w366, "DisabledEnum"=T13."Enabled" ("Disabled")) -> ()  [unwired: 1 in, 2 out]
        n222 = call "ProductString.vi"("String"="Return to production mode") -> ()  [unwired: 10 in, 1 out]
        n223 = flat-sequence {
          tunnel: w363 -> [_]
          frame #0 {
            n224 = call "IO.vi"("DO DATA"=bool[] [FALSE, FALSE, FALSE, FALSE, FALSE, FALSE, FALSE, FALSE] ("Writel_IO"), "IO Name"=string[] ["psu+   J3_1", "psu-   J3_5", "UART1_3V3  J63_1", "UART1_TX   J63_5", "UART1_RX   J63_6", "UART1_GND  J63_10", "PSU S+ J3_1", "PSU S- J3_5"], "IO?"=enum16{"DI", "DO"}."DO") -> ()  [unwired: 7 in, 2 out]
          }
        }
        "Boolean" <- w370
      }
    }
    n225 = call "Exit.vi"("Step"=enum16{"Initial", "Write", "Read"}."Read") -> ("Exit Out"=w165:bool)  [unwired: 9 in, 1 out]
    n226 = Or(x=w159, y=w165) -> (x .or. y?=w160:bool)
  }
